vi "Diff_Drive_Simulated_Hardware_Complex.vi"(7 "max_v":dbl=12.0, 8 "delta_t":dbl, 9 "b_length":dbl=0.60325, 10 "%v_bus_right":dbl, 11 "%v_bus_left":dbl) -> (0 "left_x":dbl, 1 "v_angular":dbl, 2 "x_angular":dbl, 3 "v_linear":dbl, 4 "right_x":dbl, 5 "x_linear":dbl)   [LabVIEW 2019]
panel:
  in  "Motor Velocity Constant":dbl=1069.575994
  in  "Motor Torque Constant":dbl=0.036498
  in  "Motor Resistance":dbl=0.093385214
  in  "mass":dbl=56.358852
  in  "friction":dbl
  in  "gear_ratio":dbl=0.088888
  in  "wheel_radius":dbl=0.1524
  in  "J":dbl=5.417
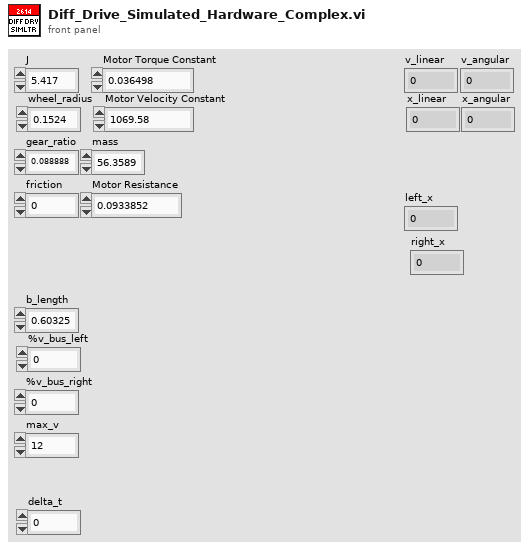
[diagram p1: front panel]
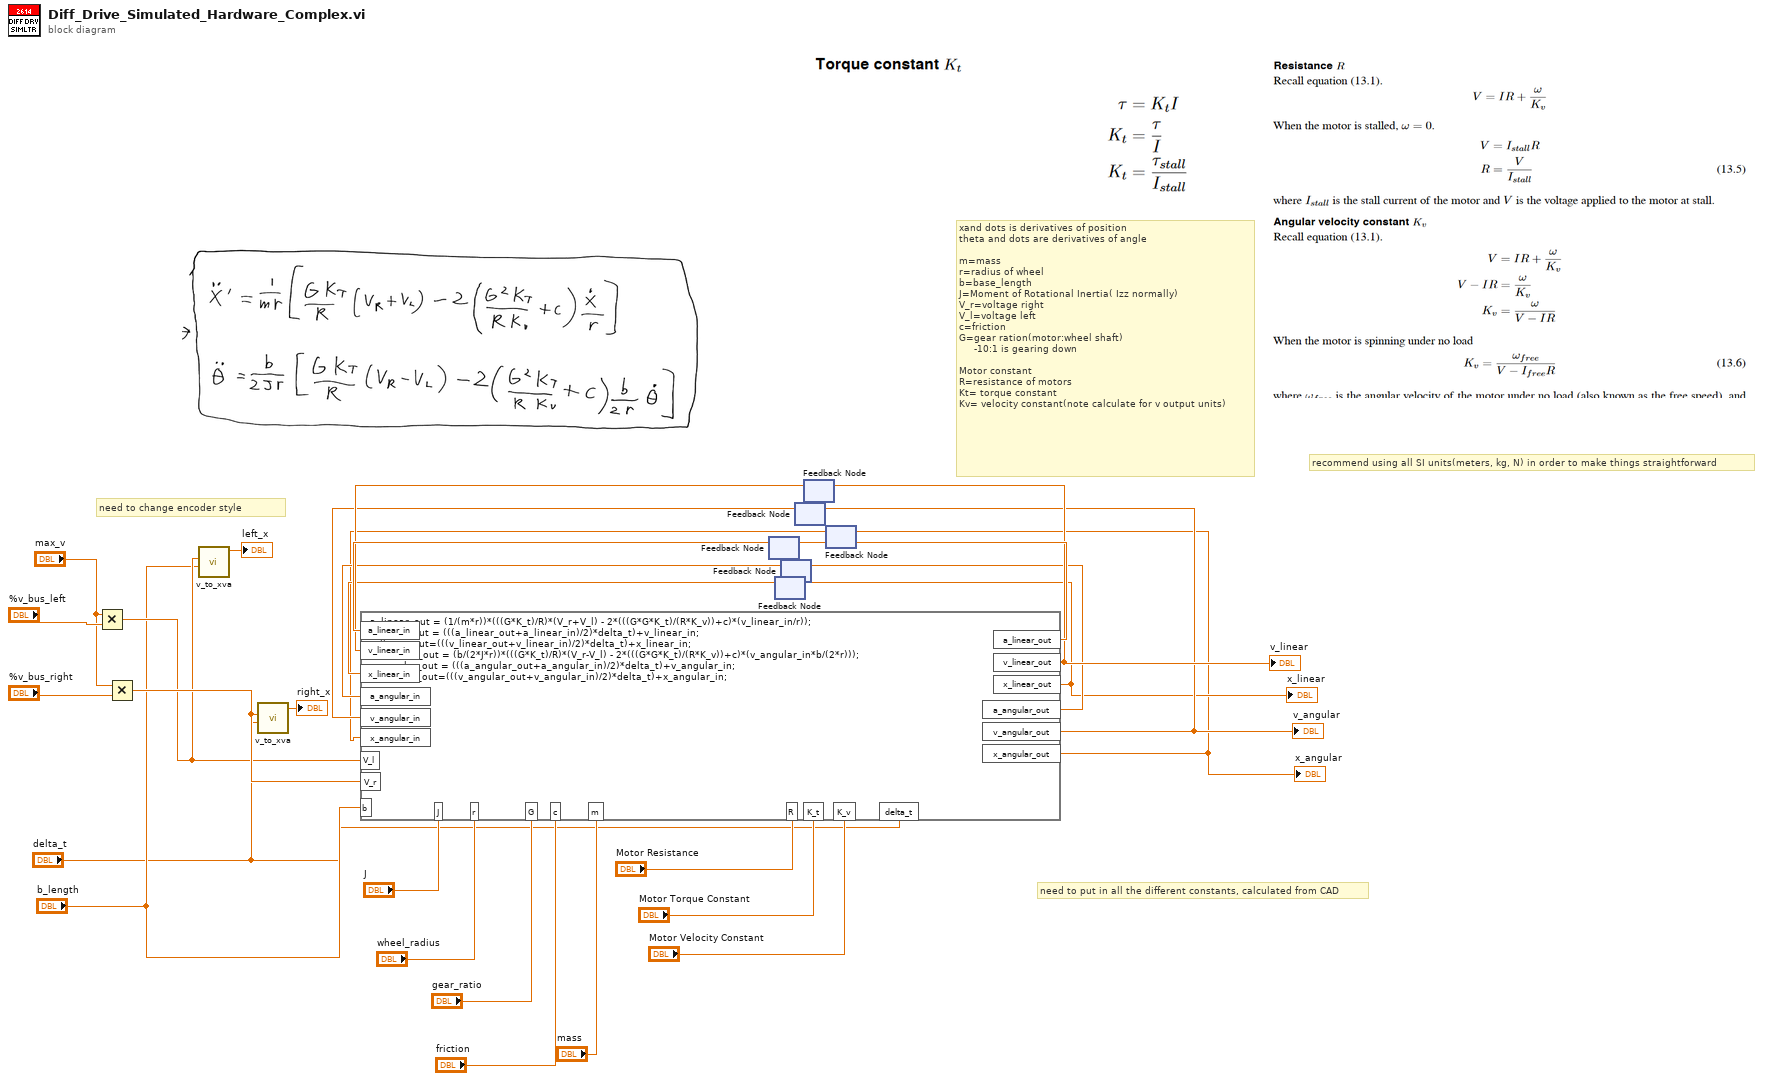
[diagram p0: block diagram]
diagram:
  # "recommend using all SI units(meters, kg, N) in order to make things straightforward"
  # "xand dots is derivatives of position\ntheta and dots are derivatives of angle\n\nm=mass\nr=radius of wheel\nb=base_length\nJ=Moment of Rotational Inertia( Izz normally)\nV_r=voltage right\nV_l=voltage left\nc=friction\nG=gear ration(motor:wheel shaft)\n     -10:1 is gearing down\n\nMotor constant\nR=resistance of motors\nKt= torque constant\nKv= velocity constant(note calculate for v output units)"
  # "need to put in all the different constants, calculated from CAD"
  # "need to change encoder style"
  n1 = Multiply(x="max_v", y="%v_bus_left") -> (x*y=w25:dbl)
  n2 = Multiply(x="max_v", y="%v_bus_right") -> (x*y=w26:dbl)
  n3 = call "v_to_xva.vi"("dt"="b_length", "v"=w25) -> ("x_out"=→"left_x":dbl)  [unwired: 7 in, 2 out]
  n4 = call "v_to_xva.vi"("dt"="delta_t", "v"=w26) -> ("x_out"=→"right_x":dbl)  [unwired: 7 in, 2 out]
  n5 = feedback #1() -> (w20:dbl)  [unwired: 1 in]
  n6 = feedback #2() -> (w17:dbl)  [unwired: 1 in]
  n7 = feedback #3() -> (w15:dbl)  [unwired: 1 in]
  n8 = feedback #4() -> (w13:dbl)  [unwired: 1 in]
  n9 = feedback #5() -> (w18:dbl)  [unwired: 1 in]
  n10 = feedback #6() -> (w12:dbl)  [unwired: 1 in]
  n11 = formula code="a_linear_out = (1/(m*r))*(((G*K_t)/R)*(V_r+V_l) - 2*(((G*G*K_t)/(R*K_v))+c)*(v_linear_in/r));\nv_linear_out = (((a_linear_out+a_linear_in)/2)*delta_t)+v_linear_in;\nx_linear_out=(((v_linear_out+v_linear_in)/2)*delta_t)+x_linear_in;\na_angular_out = (b/(2*J*r))*(((G*K_t)/R)*(V_r-V_l) - 2*(((G*G*K_t)/(R*K_v))+c)*(v_angular_in*b/(2*r)));\nv_angular_out = (((a_angular_out+a_angular_in)/2)*delta_t)+v_angular_in;\nx_angular_out=(((v_angular_out+v_angular_in)/2)*delta_t)+x_angular_in;"("V_l"=w25, "V_r"=w26, "b"="b_length", "a_linear_in"=w20, "v_linear_in"=w18, "x_linear_in"=w17, "a_angular_in"=w15, "v_angular_in"=w13, "x_angular_in"=w12, "J"="J", "r"="wheel_radius", "G"="gear_ratio", "K_v"="Motor Velocity Constant", "K_t"="Motor Torque Constant", "R"="Motor Resistance", "c"="friction", "m"="mass", "delta_t"="delta_t") -> ("a_angular_out"=w16:dbl, "a_linear_out"=w21:dbl, "v_linear_out"=w19:dbl, "x_linear_out"=w11:dbl, "v_angular_out"=w14:dbl, "x_angular_out"=w10:dbl)
  "v_linear" <- w19
  "x_linear" <- w11
  "v_angular" <- w14
  "x_angular" <- w10
  n12 = feedback-in #1(w21) -> ()
  n13 = feedback-in #2(w11) -> ()
  n14 = feedback-in #3(w16) -> ()
  n15 = feedback-in #4(w14) -> ()
  n16 = feedback-in #5(w19) -> ()
  n17 = feedback-in #6(w10) -> ()
